vi "Read.vi"(8 "error in (no error)":errorcluster, 10 "Command":T1, 11 "VISA resource name":refnum<visa-resource-name>) -> (0 "error out":errorcluster, 2 "read buffer":string, 3 "VISA resource name out":refnum<visa-resource-name>)   [LabVIEW 2020, in "Jasco UV.lvlib"]
uses:
  <instrlib>/Jasco UV/Jasco UV.lvlib
  <instrlib>/Jasco UV/Public/Data/Read Controls.ctl
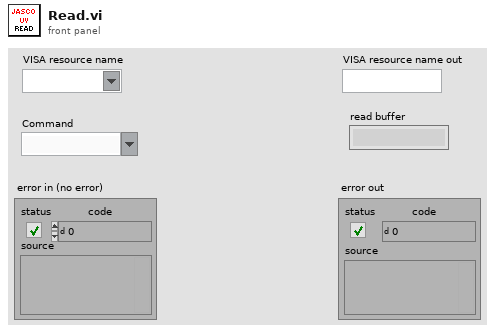
[diagram p1: front panel]
types:
  T1 = typedef "Jasco UV.lvlib/Read Controls.ctl" = string
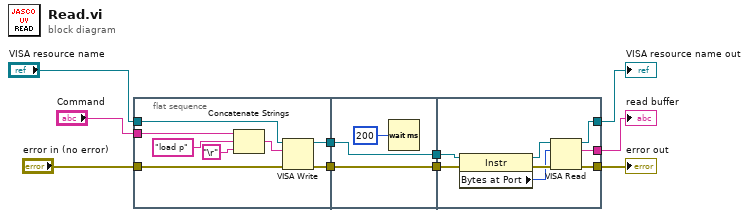
[diagram p0: block diagram]
diagram:
  n1 = flat-sequence {
    tunnel: "error in (no error)" -> [w17]
    tunnel: "VISA resource name" -> [w16]
    tunnel: [w15] -> w10
    tunnel: [w14] -> w9
    tunnel: "Command" -> [w11]
    tunnel: w10 -> [w20]
    tunnel: w9 -> [w19]
    tunnel: [w20] -> w8
    tunnel: [w19] -> w7
    tunnel: w8 -> [w28]
    tunnel: w7 -> [w26]
    tunnel: [w29] -> w4
    tunnel: [w24] -> w3
    tunnel: [w22] -> w2
    frame #0 {
      n2 = Concatenate Strings(w11, "load p" ("string"), "\r") -> (w18:string)
      n3 = VISA Write(VISA resource name=w16, write buffer=w18, error in (no error)=w17) -> (VISA resource name out=w14:refnum<visa-resource-name>, error out=w15:errorcluster)  [unwired: 1 out]
    }
    frame #1 {
      n4 = Wait (ms)(milliseconds to wait=u32 200) -> ()  [unwired: 1 out]
    }
    frame #2 {
      n5 = property class="Instr"(reference=w26, error in=w28) -> (reference out=w25:refnum<visa-resource-name>, error out=w27:errorcluster, "Bytes at Port"=w23:u32)
      n6 = VISA Read(VISA resource name=w25, byte count=w23, error in (no error)=w27) -> (VISA resource name out=w24:refnum<visa-resource-name>, read buffer=w22:string, error out=w29:errorcluster)  [unwired: 1 out]
    }
  }
  "VISA resource name out" <- w3
  "error out" <- w4
  "read buffer" <- w2
